vi "jogMotor.vi"(0 "MultiAxisController in":refnum<class "_MultiAxisController.lvclass">, 2 "axis":T2, 3 "dir":T1, 5 "error in (no error)":errorcluster) -> (14 "MultiAxisController out":refnum<class "_MultiAxisController.lvclass">, 17 "success?":bool, 18 "response":string, 19 "error out":errorcluster)   [LabVIEW 2013, in "classes.lvlib" / "_MultiAxisController.lvclass"]
doc: "Produced By:\n\n<B>Kod Integrations, LLC</B>\n4835 Marianne Drive\nMount Airy, MD 21771\nhttp://www.kodintegrations.com\nemail: info@kodintegrations.com\nphone: (240) 687-1288"
uses:
  _MultiAxisController.lvclass
  common/controls/axis.ctl
  common/controls/linear_direction.ctl
  Controller/_Controller.lvclass
  libraries/common.lvlib
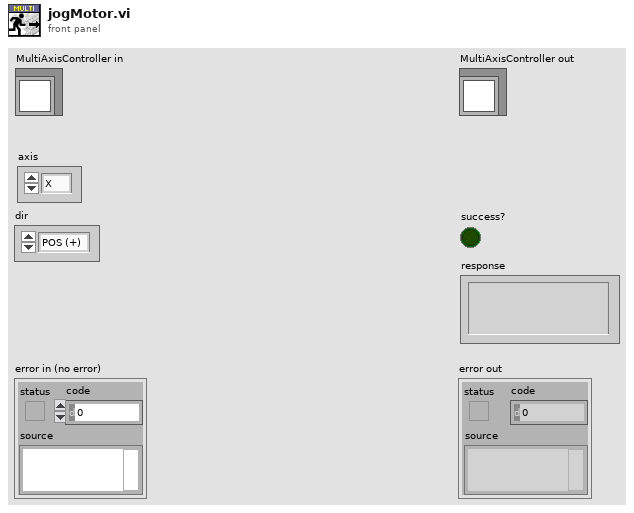
[diagram p1: front panel]
types:
  T1 = typedef "common.lvlib/linear_direction.ctl" = enum16{"POS (+)", "NEG (-)"}
  T2 = typedef "common.lvlib/axis.ctl" = enum16{"X", "Y", "Z", "U"}
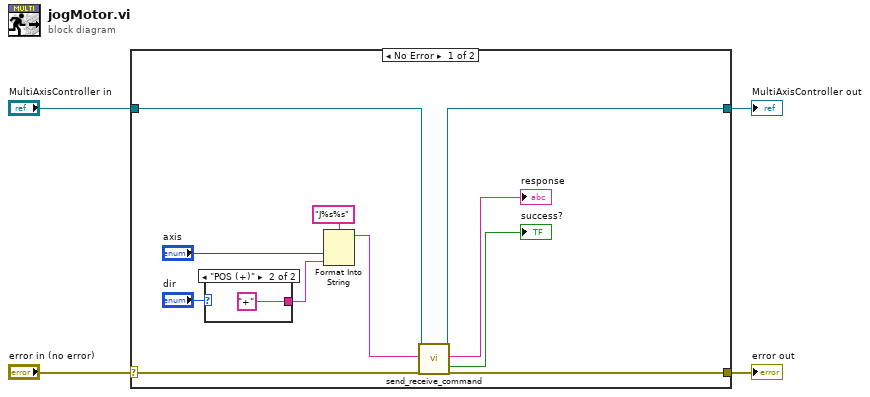
[diagram p0: block diagram]
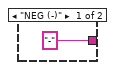
[diagram p2: hidden frame]
diagram:
  n1 = case shown="No Error" "error in (no error)" {
    selector: "error in (no error)" -> [w15 w19]
    tunnel: [w14 w19] -> w3
    tunnel: [w10 w18] -> w1
    tunnel: "MultiAxisController in" -> [w11 w18]
    frame No Error {
      n2 = case shown="\"POS (+)\"" "dir" {
        tunnel: ["-" "+"] -> w6
        frame "NEG (-)" {
        }
        frame "POS (+)" {
        }
      }
      n3 = Format Into String(format string="J%s%s", "axis", w6) -> (resulting string=w5:string)  [unwired: 2 in, 1 out]
      n4 = call "send_receive_command.vi"("reference (in)"=w11, "ASCII Command (in)"=w5, "error in (no error)"=w15) -> ("reference (out)"=w10:refnum<class "_MultiAxisController.lvclass">, "response (out)"=→"response":string, "success?"=→"success?":bool, "error out"=w14:errorcluster)  [unwired: 12 in, 1 out]
    }
    frame Error {
    }
  }
  "error out" <- w3
  "MultiAxisController out" <- w1
